vi "max-number.vi"() -> ()   [LabVIEW 2011]
panel:
  out "dPventury":dbl[unit]
  out "P2":dbl
  in  "A1/A2":dbl
  out "Density":dbl[unit]
  out "dPpitot":dbl[unit]
  out "V":dbl[unit]
  out "static_presure":dbl[unit]
  out "static_temperature":dbl[unit]
  in  "M":dbl
  in  "altitude":dbl[unit]
  out "total-temperature":dbl[unit]
  out "total-pressure":dbl[unit]
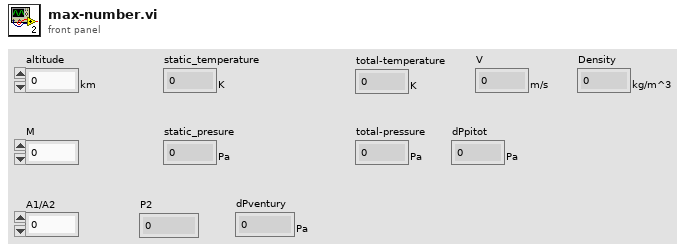
[diagram p1: front panel]
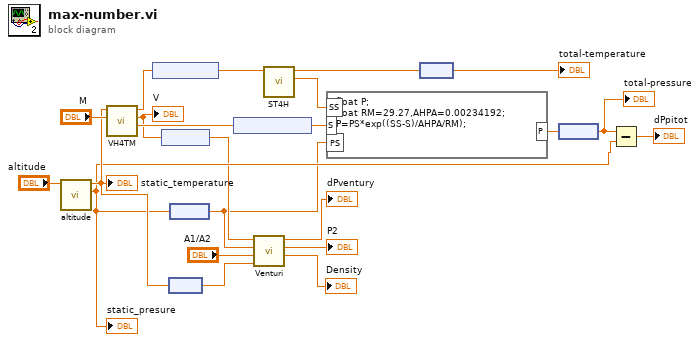
[diagram p0: block diagram]
diagram:
  n1 = call "altitude.vi"("altitude"="altitude") -> ("presure"=w10:dbl[unit], "temperature"=w19:dbl[unit])  [unwired: 9 in]
  "static_temperature" <- w19
  "static_presure" <- w10
  n2 = call "VH4TM.vi"("M"="M", "T"=w19) -> ("S"=w14:dbl[unit], "V"=w7:dbl[unit], "H"=w20:dbl[unit])  [unwired: 7 in]
  "V" <- w7
  n3 = node(w20) -> (w18:dbl)
  n4 = node(w7) -> (w6:dbl)
  n5 = node(w19) -> (w1:dbl)
  n6 = node(w10) -> (w5:dbl)
  n7 = node(w14) -> (w13:dbl)
  n8 = call "Venturi.vi"("T"=w1, "A1/A2"="A1/A2", "P"=w5, "V"=w6) -> ("Density"=→"Density":dbl[unit], "P2"=→"P2":dbl, "dPventury"=→"dPventury":dbl[unit])  [unwired: 5 in]
  n9 = call "ST4H.vi"("H"=w18) -> ("T"=w12:dbl, "S"=w17:dbl)  [unwired: 9 in]
  n10 = formula code="float P;\nfloat RM=29.27,AHPA=0.00234192;\nP=PS*exp((SS-S)/AHPA/RM);"("PS"=w5, "S"=w13, "SS"=w12) -> ("P"=w15:dbl)
  n11 = node(w17) -> (→"total-temperature":dbl[unit])
  n12 = node(w15) -> (w11:dbl[unit])
  "total-pressure" <- w11
  n13 = Subtract(x=w11, y=w10) -> (x-y=→"dPpitot":dbl[unit])
